vi "LAB6_template.vi"() -> ()   [LabVIEW 2020]
uses:
  1bb06838-fc79-41c6-bc7f-a24b9c277b47.vi
  <vilib>/Comparison/Equal/Equal Functor/Equal Functor.lvclass
panel:
  out "删除后":i32[](array[numeric])
  out "校正":i32[](array[numeric])
  out "大小":i32
  out "共几个码元出错":i32
  out "未填写学号，请正确输入":bool
  out "错码位置在":i32[](array[numeric])
  out "输出的码流":u8[](array[numeric])
  in  "12位学号":string
  in  "姓名":string
  out "接收到的字符串":string
  # "首先，请输入姓名、12位学号。\n输入错误会导致工作不正常。"
  # "汉明码编码器"
  # "汉明码译码器"
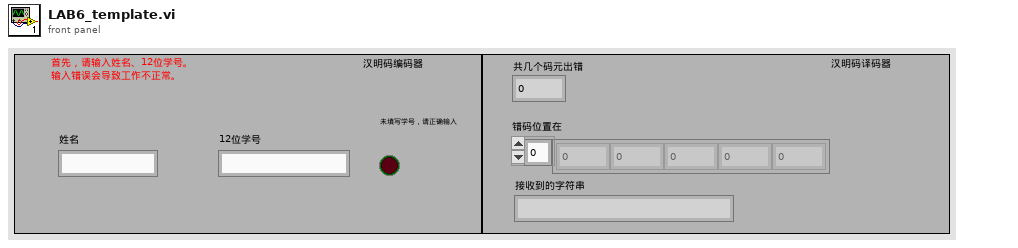
[diagram p1: front panel]
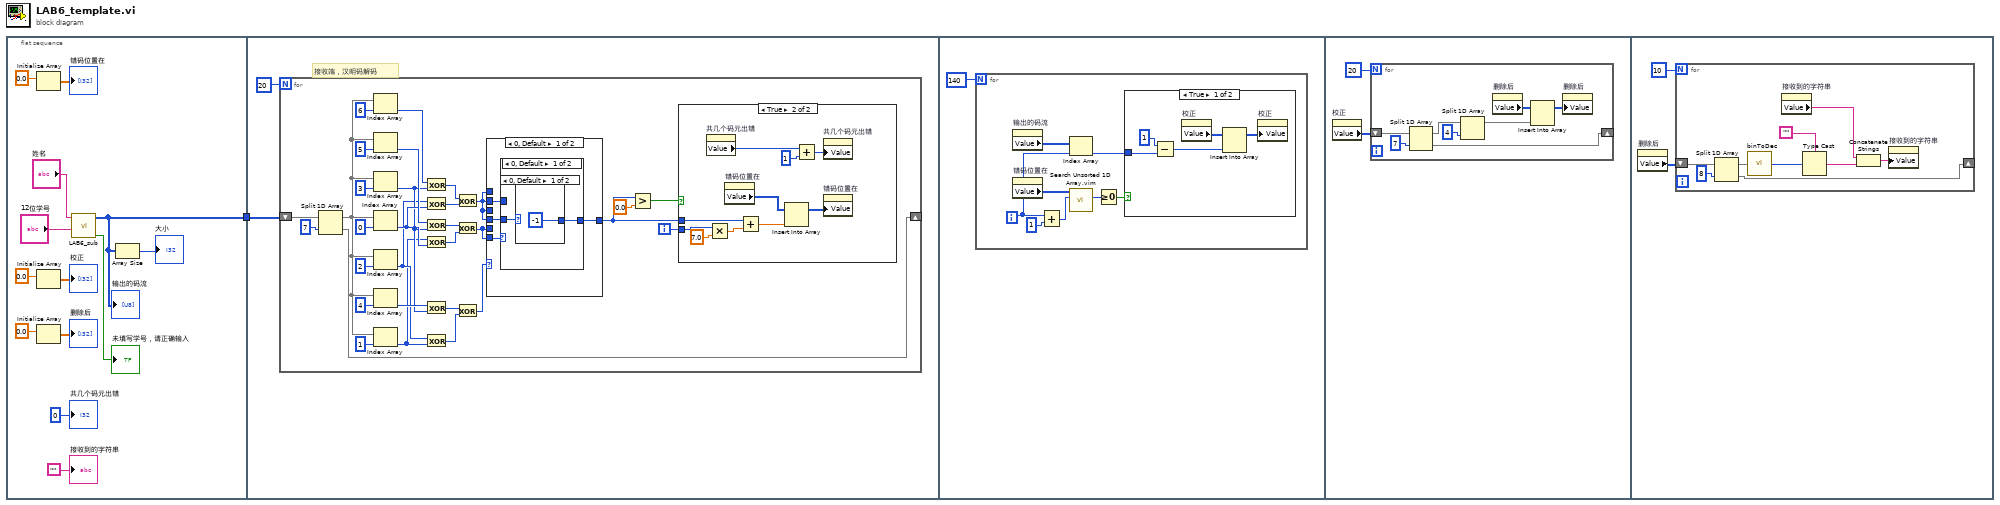
[diagram p0: block diagram]
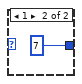
[diagram p3: hidden frame]
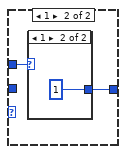
[diagram p4: hidden frame]
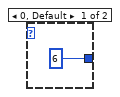
[diagram p5: hidden frame]
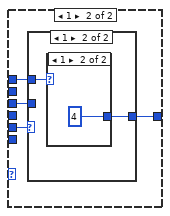
[diagram p6: hidden frame]
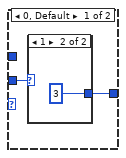
[diagram p7: hidden frame]
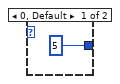
[diagram p8: hidden frame]
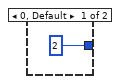
[diagram p9: hidden frame]
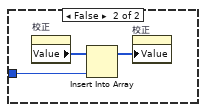
[diagram p10: hidden frame]
diagram:
  n1 = flat-sequence {
    tunnel: [w7] -> w1
    tunnel: w1 -> [w16]
    frame #0 {
      n2 = Initialize Array(0.0 ("element")) -> (→"错码位置在":dbl[])  [unwired: 1 in]
      n3 = Initialize Array(0.0 ("element")) -> (→"校正":dbl[])  [unwired: 1 in]
      n4 = Initialize Array(0.0 ("element")) -> (→"删除后":dbl[])  [unwired: 1 in]
      n5 = call "LAB6_sub.vi"("12位学号"="12位学号", "姓名"="姓名") -> ("未输入学号"=→"未填写学号，请正确输入":bool, "输出的码流"=w7:u8[])  [unwired: 8 in]
      "输出的码流" <- w7
      n6 = Array Size(array=w7) -> (size(s)=→"大小":i32)
      "共几个码元出错" <- 0 ("共几个码元出错")
      "接收到的字符串" <- ""
    }
    frame #1 {
      # "接收端，汉明码解码"
      n7 = for {
        N: 20 -> [_]
        shift-right: [w45] -> _
        shift-left: w16 -> [w46]
        i -> [w21]
        n8 = Split 1D Array(array=w46, index=7) -> (first subarray=w37:u8[], second subarray=w45:u8[])
        n9 = Index Array(array=w37, index=6) -> (element=w30:u8)
        n10 = Index Array(array=w37, index=5) -> (element=w29:u8)
        n11 = Index Array(array=w37, index=3) -> (element=w26:u8)
        n12 = Index Array(array=w37, index=0) -> (element=w28:u8)
        n13 = Index Array(array=w37, index=2) -> (element=w25:u8)
        n14 = Index Array(array=w37, index=4) -> (element=w27:u8)
        n15 = Index Array(array=w37, index=1) -> (element=w24:u8)
        n16 = Exclusive Or(1:w26, 2:w30) -> (0:w33:u8)
        n17 = Exclusive Or(1:w28, 2:w25) -> (0:w35:u8)
        n18 = Exclusive Or(1:w26, 2:w29) -> (0:w36:u8)
        n19 = Exclusive Or(1:w28, 2:w24) -> (0:w34:u8)
        n20 = Exclusive Or(1:w26, 2:w27) -> (0:w31:u8)
        n21 = Exclusive Or(1:w24, 2:w25) -> (0:w32:u8)
        n22 = Exclusive Or(1:w35, 2:w33) -> (0:w19:u8)
        n23 = Exclusive Or(1:w34, 2:w36) -> (0:w18:u8)
        n24 = Exclusive Or(1:w32, 2:w31) -> (0:w17:u8)
        n25 = case shown="0, Default" w17 {
          tunnel: w18 -> [_ w73]
          tunnel: w19 -> [_ w72]
          tunnel: w19 -> [_ w71]
          tunnel: w18 -> [w61 _]
          tunnel: w19 -> [w60 _]
          tunnel: w19 -> [w59 _]
          tunnel: [w58 w70] -> w20
          frame 0, Default {
            n26 = case shown="0, Default" w61 {
              tunnel: w60 -> [_ w67]
              tunnel: w59 -> [w63 _]
              tunnel: [w62 w66] -> w58
              frame 0, Default {
                n27 = case shown="0, Default" w63 {
                  tunnel: [-1 7] -> w62
                  frame 0, Default {
                  }
                  frame 1 {
                  }
                }
              }
              frame 1 {
                n28 = case shown="1" w67 {
                  tunnel: [6 1] -> w66
                  frame 0, Default {
                  }
                  frame 1 {
                  }
                }
              }
            }
          }
          frame 1 {
            n29 = case shown="1" w73 {
              tunnel: w72 -> [_ w79]
              tunnel: w71 -> [w75 _]
              tunnel: [w74 w78] -> w70
              frame 0, Default {
                n30 = case shown="1" w75 {
                  tunnel: [5 3] -> w74
                  frame 0, Default {
                  }
                  frame 1 {
                  }
                }
              }
              frame 1 {
                n31 = case shown="1" w79 {
                  tunnel: [2 4] -> w78
                  frame 0, Default {
                  }
                  frame 1 {
                  }
                }
              }
            }
          }
        }
        n32 = Greater?(x=w20, y=0.0) -> (0:w22:bool)
        n33 = case shown="True" w22 {
          tunnel: w21 -> [_ w55]
          tunnel: w20 -> [_ w54]
          frame False {
          }
          frame True {
            n34 = property on="共几个码元出错" class="DigNum (strict)"() -> ("Value"=w52:i32)  [unwired: 2 in, 2 out]
            n35 = Multiply(x=w55, y=7.0) -> (x*y=w57:dbl)
            n36 = property on="错码位置在" class="Arr (strict)"() -> ("Value"=w53:i32[])  [unwired: 2 in, 2 out]
            n37 = Add(x=w54, y=w57) -> (x+y=w48:dbl)
            n38 = Insert Into Array(array=w53, new element=w48) -> (w49:i32[])  [unwired: 1 in]
            n39 = Add(x=w52, y=1) -> (x+y=w50:i32)
            n40 = property on="共几个码元出错" class="DigNum (strict)"("Value"=w50) -> ()  [unwired: 2 in, 2 out]
            n41 = property on="错码位置在" class="Arr (strict)"("Value"=w49) -> ()  [unwired: 2 in, 2 out]
          }
        }
      }
    }
    frame #2 {
      n42 = for {
        N: 140 -> [_]
        i -> [w88]
        n43 = property on="输出的码流" class="Arr (strict)"() -> ("Value"=w90:u8[])  [unwired: 2 in, 2 out]
        n44 = property on="错码位置在" class="Arr (strict)"() -> ("Value"=w89:i32[])  [unwired: 2 in, 2 out]
        n45 = Add(x=w88, y=1) -> (x+y=w86:i32)
        n46 = Index Array(array=w90, index=w88) -> (element=w85:u8)
        n47 = call "Search Unsorted 1D Array.vim"("element"=w86, "unsorted 1D array"=w89) -> ("index of element"=w84:i32)  [unwired: 9 in]
        n48 = Greater Or Equal To 0?(x=w84) -> (x >= 0?=w83:bool)
        n49 = case shown="True" w83 {
          tunnel: w85 -> [w94 w97]
          frame True {
            n50 = Subtract(x=u8 1, y=w94) -> (x-y=w91:u8)
            n51 = property on="校正" class="Arr (strict)"() -> ("Value"=w92:i32[])  [unwired: 2 in, 2 out]
            n52 = Insert Into Array(array=w92, new element=w91) -> (w93:i32[])  [unwired: 1 in]
            n53 = property on="校正" class="Arr (strict)"("Value"=w93) -> ()  [unwired: 2 in, 2 out]
          }
          frame False {
            n54 = property on="校正" class="Arr (strict)"() -> ("Value"=w98:i32[])  [unwired: 2 in, 2 out]
            n55 = Insert Into Array(array=w98, new element=w97) -> (w96:i32[])  [unwired: 1 in]
            n56 = property on="校正" class="Arr (strict)"("Value"=w96) -> ()  [unwired: 2 in, 2 out]
          }
        }
      }
    }
    frame #3 {
      n57 = property on="校正" class="Arr (strict)"() -> ("Value"=w99:i32[])  [unwired: 2 in, 2 out]
      n58 = for {
        N: 20 -> [_]
        shift-right: [w106] -> _
        shift-left: w99 -> [w107]
        n59 = Split 1D Array(array=w107, index=7) -> (first subarray=w105:i32[], second subarray=w106:i32[])
        n60 = Split 1D Array(array=w105, index=4) -> (first subarray=w102:i32[])  [unwired: 1 out]
        n61 = property on="删除后" class="Arr (strict)"() -> ("Value"=w103:i32[])  [unwired: 2 in, 2 out]
        n62 = Insert Into Array(array=w103, new element=w102) -> (w101:i32[])  [unwired: 1 in]
        n63 = property on="删除后" class="Arr (strict)"("Value"=w101) -> ()  [unwired: 2 in, 2 out]
      }
    }
    frame #4 {
      n64 = property on="删除后" class="Arr (strict)"() -> ("Value"=w109:i32[])  [unwired: 2 in, 2 out]
      n65 = for {
        N: 10 -> [_]
        shift-right: [w117] -> _
        shift-left: w109 -> [w118]
        n66 = Split 1D Array(array=w118, index=8) -> (first subarray=w116:i32[], second subarray=w117:i32[])
        n67 = call "binToDec.vi"("Array 2"=w116) -> ("output"=w111:i32)
        n68 = property on="接收到的字符串" class="Str"() -> ("Value"=w112:string)  [unwired: 2 in, 2 out]
        n69 = Type Cast(type="", x=w111) -> (*(type *) &x=w113:string)
        n70 = Concatenate Strings(w112, w113) -> (w114:string)
        n71 = property on="接收到的字符串" class="Str"("Value"=w114) -> ()  [unwired: 2 in, 2 out]
      }
    }
  }
